vi "ReadExEventNoLoop.vi"() -> ()   [LabVIEW 2015]
uses:
  GPS_Driver_Global.vi
panel:
  in  "Path to FITS Header File":path=path "C:/Users/Public/Documents/SI Image SGL II -/Other Parameters.txt"
  out "# Entries After":i16
  in  "# Entries Before":i16
  out "Close Min":u32
  out "Close Maj":u32
  out "Open Min":u32
  out "Open Maj":u32
  out "error out":errorcluster
  in  "error in (no error)":errorcluster
  # "Major UNIX Time:"
  # "Minor UNIX Time:"
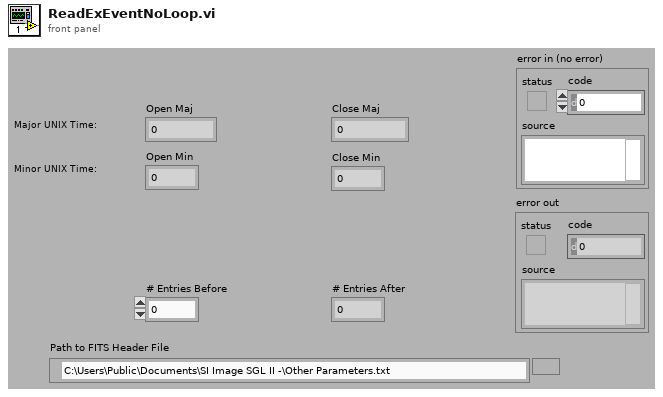
[diagram p1: front panel]
types:
  T1 = cluster{"Close":cluster{"Time":string, "Error":string}, "Open":cluster{"Time":string, "Error":string}, "Date":cluster{"Date":string, "Error":string}}
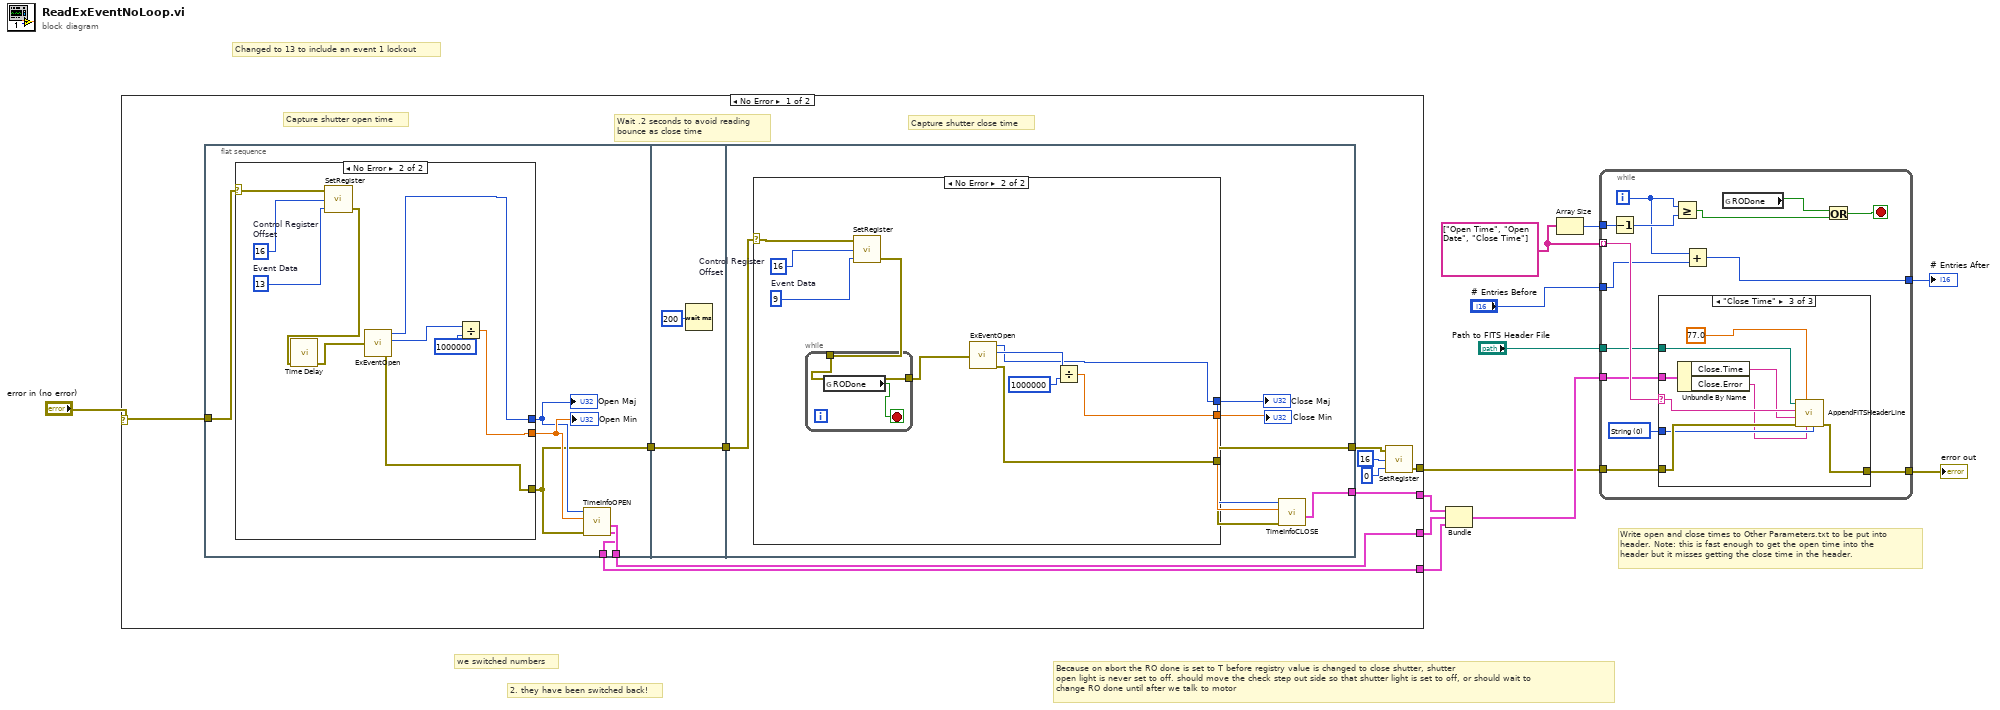
[diagram p0: block diagram]
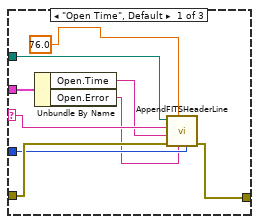
[diagram p2: hidden frame]
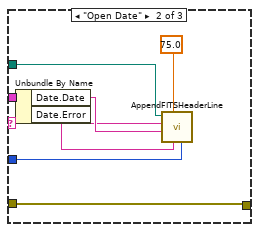
[diagram p3: hidden frame]
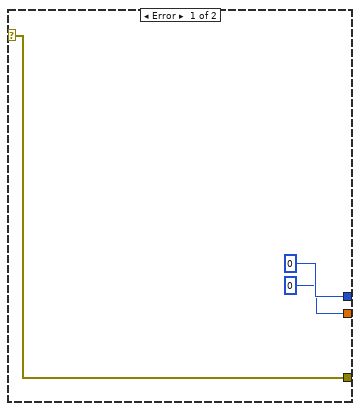
[diagram p4: hidden frame]
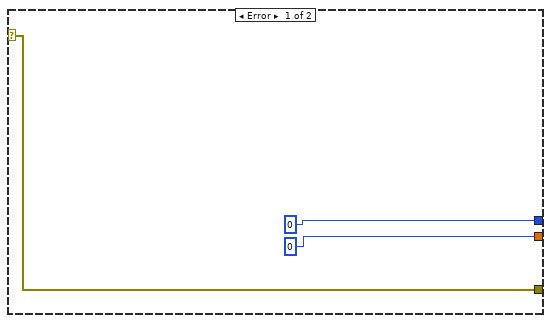
[diagram p5: hidden frame]
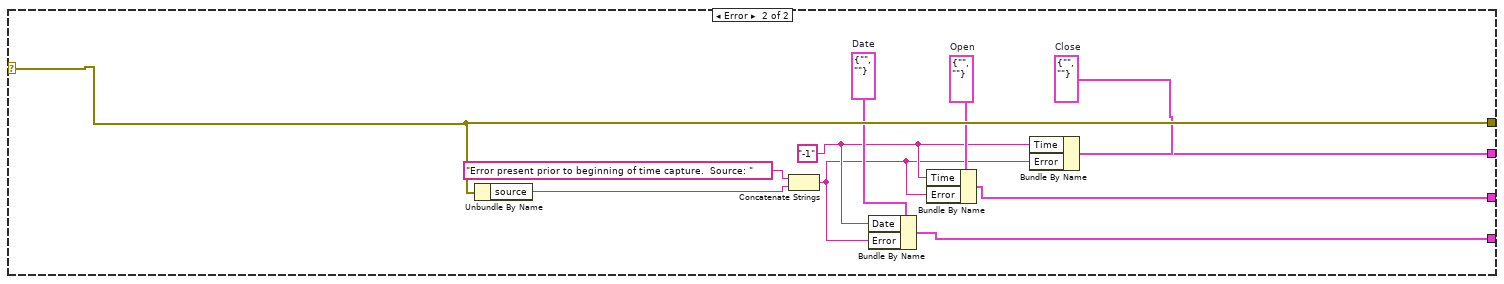
[diagram p6: hidden frame]
diagram:
  w12 = string[] ["Open Time", "Open Date", "Close Time"]
  # "Changed to 13 to include an event 1 lockout"
  # "Because on abort the RO done is set to T before registry value is changed to close shutter, shutter\nopen light is never set to off. should move the check step out side so that shutter light is set to off, or should wait to \nchange RO done until after we talk to motor"
  # "2. they have been switched back!"
  # "we switched numbers"
  # "Write open and close times to Other Parameters.txt to be put into\nheader. Note: this is fast enough to get the open time into the \nheader but it misses getting the close time in the header."
  n1 = case shown="No Error" "error in (no error)" {
    selector: "error in (no error)" -> [w13 w74]
    tunnel: [w20 w74] -> w7
    tunnel: [w19 w67] -> w8
    tunnel: [w18 w70] -> w9
    tunnel: [w14 w68] -> w1
    frame No Error {
      # "Capture shutter close time"
      # "Wait .2 seconds to avoid reading \nbounce as close time"
      # "Capture shutter open time"
      n2 = flat-sequence {
        tunnel: w13 -> [w26]
        tunnel: [w25] -> w19
        tunnel: [w24] -> w16
        tunnel: [w23] -> w14
        tunnel: [w42] -> w17
        tunnel: w16 -> [w42]
        tunnel: [w46] -> w18
        tunnel: w17 -> [w45]
        tunnel: [w44] -> w15
        frame #0 {
          n3 = case shown="No Error" w26 {
            selector: w26 -> [w29 w37]
            tunnel: [0 w34] -> w28
            tunnel: [w29 w36] -> w24
            tunnel: [0 w35] -> w27
            frame Error {
            }
            frame No Error {
              w40 = 13  # Event Data
              w41 = 16  # Control Register Offset
              n4 = call "SetRegister.vi"("Data"=w40, "Offset"=w41, "error in (no error)"=w37) -> ("error out"=w33:errorcluster)  [unwired: 2 in]
              n5 = call "Time Delay"("error in (no error)"=w33) -> ("error out"=w32:errorcluster)  [unwired: 10 in]
              n6 = call "ExEventOpen.vi"("error in (no error)"=w32) -> ("Major Time"=w35:u32, "Minor Time"=w39:u32, "error out"=w36:errorcluster)  [unwired: 1 in]
              n7 = Divide(x=w39, y=1000000) -> (x/y=w34:dbl)
            }
          }
          "Open Min" <- w28
          "Open Maj" <- w27
          n8 = call "TimeInfoOPEN.vi"("error in (no error)"=w24, "Minor Time"=w28, "Major Time"=w27) -> ("Date"=w23:cluster{"Date":string, "Error":string}, "Open"=w25:cluster{"Time":string, "Error":string})  [unwired: 6 in]
        }
        frame #1 {
          n9 = Wait (ms)(milliseconds to wait=200) -> ()  [unwired: 1 out]
        }
        frame #2 {
          n10 = case shown="No Error" w45 {
            selector: w45 -> [w49 w57]
            tunnel: [0 w53] -> w48
            tunnel: [w49 w52] -> w44
            tunnel: [0 w54] -> w47
            frame Error {
            }
            frame No Error {
              w60 = 9  # Event Data
              w61 = 16  # Control Register Offset
              n11 = call "SetRegister.vi"("Data"=w60, "Offset"=w61, "error in (no error)"=w57) -> ("error out"=w56:errorcluster)  [unwired: 2 in]
              n12 = while {
                tunnel: [w62] -> w55
                tunnel: w56 -> [w62]
                stop <- w63 stop-if-true
                n13 = global read "GPS_Driver_Global.vi" "RODone"() -> (w63:bool)
              }
              n14 = call "ExEventOpen.vi"("error in (no error)"=w55) -> ("Major Time"=w54:u32, "Minor Time"=w59:u32, "error out"=w52:errorcluster)  [unwired: 1 in]
              n15 = Divide(x=w59, y=1000000) -> (x/y=w53:dbl)
            }
          }
          "Close Maj" <- w47
          "Close Min" <- w48
          n16 = call "TimeInfoCLOSE.vi"("error in (no error)"=w44, "Minor Time"=w48, "Major Time"=w47) -> ("Close"=w46:cluster{"Time":string, "Error":string})  [unwired: 7 in]
        }
      }
      n17 = call "SetRegister.vi"("Data"=0, "Offset"=16, "error in (no error)"=w15) -> ("error out"=w20:errorcluster)  [unwired: 2 in]
    }
    frame Error {
      w66 = cluster{"Date":string, "Error":string} {"Date"="", "Error"=""}  # Date
      w71 = cluster{"Time":string, "Error":string} {"Time"="", "Error"=""}  # Close
      w69 = cluster{"Time":string, "Error":string} {"Time"="", "Error"=""}  # Open
      w65 = "-1"
      n18 = Unbundle By Name(w74) -> ("source"=w72:string)
      n19 = Concatenate Strings("Error present prior to beginning of time capture.  Source: ", w72) -> (w64:string)
      n20 = Bundle By Name(cluster=w66, "Date"=w65, "Error"=w64) -> (w68:cluster{"Date":string, "Error":string})
      n21 = Bundle By Name(cluster=w69, "Time"=w65, "Error"=w64) -> (w67:cluster{"Time":string, "Error":string})
      n22 = Bundle By Name(cluster=w71, "Time"=w65, "Error"=w64) -> (w70:cluster{"Time":string, "Error":string})
    }
  }
  n23 = Bundle("Close"=w9, "Open"=w8, "Date"=w1) -> (w11:T1)  [unwired: 1 in]
  n24 = Array Size(array=w12) -> (size(s)=w5:i32)
  n25 = while {
    tunnel: w7 -> [w88]
    tunnel: w12 -> [w86] mode=indexing
    tunnel: w5 -> [w85]
    tunnel: "# Entries Before" -> [w83]
    tunnel: w11 -> [w81]
    tunnel: "Path to FITS Header File" -> [w80]
    tunnel: [w79] -> w10
    tunnel: [w75] -> w3
    i -> [w82]
    stop <- w77 stop-if-true
    w84 = u16 0 items=["String", "Numeric", "Boolean"]
    n26 = Decrement(x=w85) -> (x-1=w87:i32)
    n27 = case shown="\"Close Time\"" w86 {
      selector: w86 -> [w95 w100 w113]
      tunnel: w88 -> [w97 w99 w114]
      tunnel: w84 -> [w96 w104 w112]
      tunnel: w81 -> [w92 w103 w109]
      tunnel: w80 -> [w94 w105 w110]
      tunnel: [w93 w99 w111] -> w79
      frame "Open Time", Default {
        n28 = Unbundle By Name(w92) -> ("Open.Time"=w91:string, "Open.Error"=w90:string)
        n29 = call "AppendFITSHeaderLine.vi"("Entry Type"=w96, "Comment"=w90, "Entry #"=76.0, "error in (no error)"=w97, "Element Value"=w91, "Element Name"=w95, "file path (dialog if empty)"=w94) -> ("error out"=w93:errorcluster)  [unwired: 3 in]
      }
      frame "Open Date" {
        n30 = Unbundle By Name(w103) -> ("Date.Date"=w102:string, "Date.Error"=w101:string)
        n31 = call "AppendFITSHeaderLine.vi"("Entry Type"=w104, "Comment"=w101, "Entry #"=75.0, "Element Value"=w102, "Element Name"=w100, "file path (dialog if empty)"=w105) -> ()  [unwired: 4 in, 1 out]
      }
      frame "Close Time" {
        n32 = Unbundle By Name(w109) -> ("Close.Time"=w108:string, "Close.Error"=w107:string)
        n33 = call "AppendFITSHeaderLine.vi"("Entry Type"=w112, "Comment"=w107, "Entry #"=77.0, "error in (no error)"=w114, "Element Value"=w108, "Element Name"=w113, "file path (dialog if empty)"=w110) -> ("error out"=w111:errorcluster)  [unwired: 3 in]
      }
    }
    n34 = Greater Or Equal?(x=w82, y=w87) -> (x >= y?=w78:bool)
    n35 = Add(x=w82, y=w83) -> (x+y=w75:i32)
    n36 = global read "GPS_Driver_Global.vi" "RODone"() -> (w76:bool)
    n37 = Or(x=w76, y=w78) -> (x .or. y?=w77:bool)
  }
  "error out" <- w10
  "# Entries After" <- w3
